vi "Save Scan to File.vi"(8 "error in":errorcluster, 9 "Tree Map in":T1, 11 "Path":path) -> (0 "error out":errorcluster, 1 "Tree Map Out":T1)   [LabVIEW 2019, in "Panther Dashboard.lvlib"]
uses:
  Panther Dashboard.lvlib
  <vilib>/National Instruments/Tree Map/Tree Map Data.ctl
  <vilib>/National Instruments/Tree Map/Tree Map.lvlib
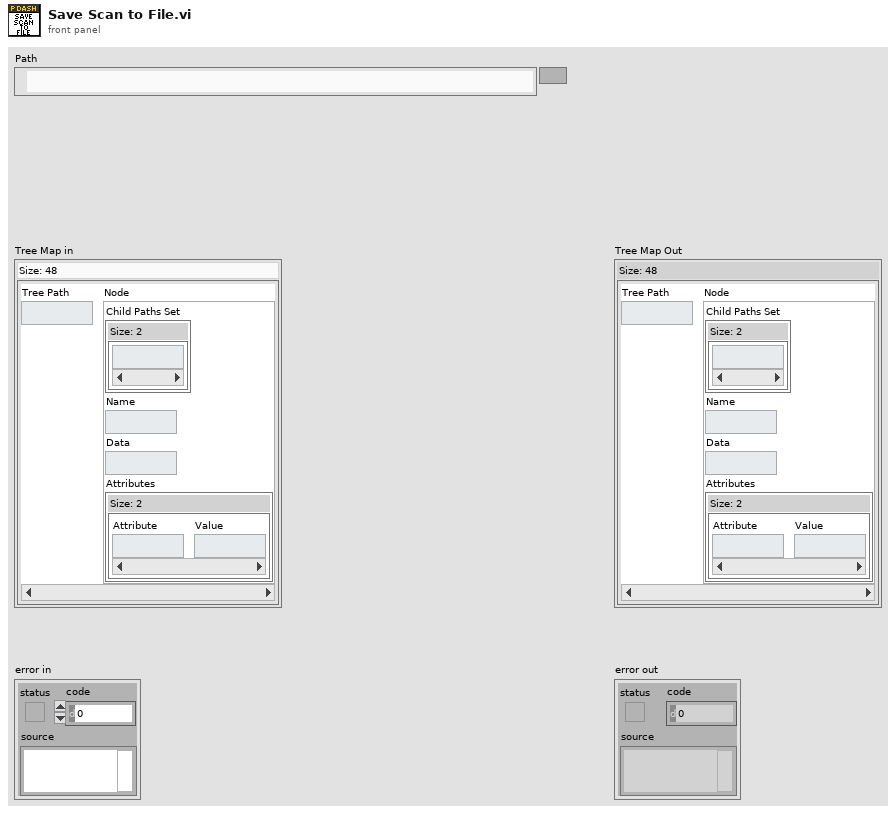
[diagram p1: front panel]
types:
  T1 = typedef "Tree Map.lvlib/Tree Map Data.ctl" = map{string, cluster{"Child Paths Set":set{string}, "Name":string, "Data":string, "Attributes":map{string, string}}}
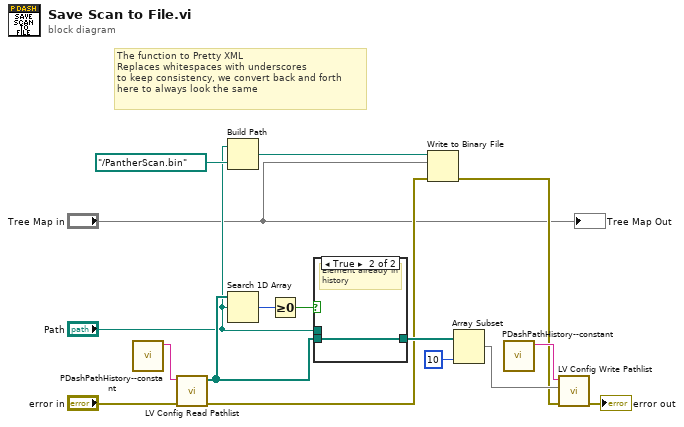
[diagram p0: block diagram]
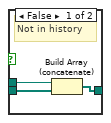
[diagram p2: hidden frame]
diagram:
  # "The function to Pretty XML\nReplaces whitespaces with underscores\nto keep consistency, we convert back and forth\nhere to always look the same"
  n1 = call "PDashPathHistory--constant.vi"() -> ("PDashPathHistory"=w13:string)  [unwired: 11 in]
  n2 = call <resource>:"LV Config Read Pathlist.vi"("error in"="error in", "key"=w13) -> ("error out"=w3:errorcluster, "value"=w11:path[])  [unwired: 3 in, 1 out]
  n3 = Build Path(base path="Path", name or relative path=path "../PantherScan.bin") -> (appended path=w9:path)
  n4 = Search 1D Array(1D array=w11, element="Path") -> (index of element=w12:i32)  [unwired: 1 in]
  n5 = Greater Or Equal To 0?(x=w12) -> (x >= 0?=w10:bool)
  n6 = case shown="True" w10 {
    tunnel: w11 -> [w19 w20]
    tunnel: [w17 w20] -> w8
    tunnel: "Path" -> [w18 _]
    frame False {
      # "Not in history"
      n7 = Build Array (concatenate)(w18, w19) -> (w17:path[])
    }
    frame True {
      # "Element already in history"
    }
  }
  n8 = Write to Binary File(file (use dialog)=w9, data="Tree Map in", error in=w3) -> (error out=w2:errorcluster)  [unwired: 3 in, 2 out]
  n9 = Array Subset(array=w8, length=10) -> (w7:path[])  [unwired: 1 in]
  n10 = call "PDashPathHistory--constant.vi"() -> ("PDashPathHistory"=w4:string)  [unwired: 11 in]
  n11 = call <resource>:"LV Config Write Pathlist.vi"("error in (no error)"=w2, "value"=w7, "key"=w4) -> ("error out"=→"error out":errorcluster)  [unwired: 4 in]
  "Tree Map Out" <- "Tree Map in"
